vi "test_wpt_sim.vi"() -> ()   [LabVIEW 2019]
uses:
  Ctrl/waypoint_buf.ctl
panel:
  out "size(s)":i32=8
  out "XY Graph":cluster{cluster{dbl, dbl}[]}[](graph)=[{[{7.857142857142858, 2.6530612244897958}]}, {[{-1.0, 1.5}, {-0.9042553191489362, 1.5319148936170213}, {-0.8085106382978724, 1.5638297872340425}, {-0.7127659574468085, 1.5957446808510638}, {-0.6170212765957447, 1.627659574468085}, {-0.5212765957446809, 1.6595744680851063}, {-0.42553191489361697, 1.6914893617021276}, {-0.32978723404255317, 1.7234042553191489}, {-0.23404255319148937, 1.7553191489361701}, {-0.13829787234042556, 1.7872340425531914}, {-0.042553191489361764, 1.8191489361702127}, {0.05319148936170204, 1.851063829787234}, {0.14893617021276606, 1.8829787234042552}, {0.24468085106382986, 1.9148936170212765}, {0.34042553191489366, 1.9468085106382977}, {0.43617021276595747, 1.978723404255319}, {0.5319148936170213, 2.0106382978723403}, {0.6276595744680851, 2.0425531914893615}, {0.7234042553191489, 2.074468085106383}, {0.8191489361702127, 2.106382978723404}, {0.9148936170212765, 2.1382978723404253}, {1.0106382978723403, 2.1702127659574466}, {1.106382978723404, 2.202127659574468}, {1.2021276595744679, 2.234042553191489}, {1.2978723404255321, 2.2659574468085104}, {1.393617021276596, 2.297872340425532}, {1.4893617021276597, 2.329787234042553}, {1.5851063829787235, 2.3617021276595747}, {1.6808510638297873, 2.3936170212765955}, {1.7765957446808511, 2.425531914893617}, {1.872340425531915, 2.457446808510638}, {1.9680851063829787, 2.4893617021276597}, {2.0638297872340425, 2.5212765957446805}, {2.1595744680851063, 2.5531914893617023}, {2.25531914893617, 2.585106382978723}, {2.351063829787234, 2.617021276595745}, {2.4468085106382977, 2.6489361702127656}, {2.5425531914893615, 2.6808510638297873}, {2.6382978723404253, 2.712765957446808}, {2.734042553191489, 2.74468085106383}, {2.829787234042553, 2.7765957446808507}, {2.925531914893617, 2.8085106382978724}, {3.0212765957446805, 2.840425531914893}, {3.117021276595745, 2.872340425531915}, {3.212765957446808, 2.9042553191489358}, {3.3085106382978724, 2.9361702127659575}, {3.4042553191489358, 2.9680851063829783}, {3.5, 3.0}, {3.59375, 2.96875}, {3.6875, 2.9375}, {3.78125, 2.90625}, {3.875, 2.875}, {3.96875, 2.84375}, {4.0625, 2.8125}, {4.15625, 2.78125}, {4.25, 2.75}, {4.34375, 2.71875}, {4.4375, 2.6875}, {4.53125, 2.65625}, {4.625, 2.625}, {4.71875, 2.59375}, {4.8125, 2.5625}, {4.90625, 2.53125}, {5.0, 2.5}, {5.096153846153846, 2.5288461538461537}, {5.1923076923076925, 2.5576923076923075}, {5.288461538461538, 2.5865384615384617}, {5.384615384615385, 2.6153846153846154}, {5.480769230769231, 2.644230769230769}, {5.576923076923077, 2.673076923076923}, {5.673076923076923, 2.701923076923077}, {5.769230769230769, 2.730769230769231}, {5.865384615384615, 2.7596153846153846}, {5.961538461538462, 2.7884615384615383}, {6.0576923076923075, 2.8173076923076925}, {6.153846153846154, 2.8461538461538463}, {6.25, 2.875}, {6.346153846153847, 2.9038461538461537}, {6.4423076923076925, 2.9326923076923075}, {6.538461538461538, 2.9615384615384617}, {6.634615384615385, 2.9903846153846154}, {6.730769230769231, 3.019230769230769}, {6.826923076923077, 3.0480769230769234}, {6.923076923076923, 3.076923076923077}, {7.019230769230769, 3.105769230769231}, {7.115384615384615, 3.1346153846153846}, {7.211538461538462, 3.1634615384615383}, {7.307692307692308, 3.1923076923076925}, {7.403846153846154, 3.2211538461538463}, {7.5, 3.25}, {7.596153846153847, 3.2788461538461537}, {7.6923076923076925, 3.3076923076923075}, {7.788461538461538, 3.3365384615384617}, {7.884615384615385, 3.3653846153846154}, {7.980769230769231, 3.394230769230769}, {8.076923076923077, 3.4230769230769234}, {8.173076923076923, 3.451923076923077}, {8.26923076923077, 3.480769230769231}, {8.365384615384615, 3.5096153846153846}, {8.461538461538462, 3.5384615384615383}, {8.557692307692308, 3.5673076923076925}, {8.653846153846153, 3.5961538461538463}, {8.75, 3.625}, {8.846153846153847, 3.653846153846154}, {8.942307692307693, 3.6826923076923075}, {9.038461538461538, 3.7115384615384617}, {9.134615384615385, 3.7403846153846154}, {9.23076923076923, 3.769230769230769}, {9.326923076923077, 3.7980769230769234}, {9.423076923076923, 3.826923076923077}, {9.51923076923077, 3.855769230769231}, {9.615384615384617, 3.8846153846153846}, {9.711538461538462, 3.9134615384615383}, {9.807692307692308, 3.9423076923076925}, {9.903846153846153, 3.9711538461538463}, {10.0, 4.0}, {10.06, 3.92}, {10.12, 3.84}, {10.18, 3.76}, {10.24, 3.68}, {10.3, 3.6}, {10.36, 3.52}, {10.42, 3.44}, {10.48, 3.36}, {10.54, 3.2800000000000002}, {10.6, 3.2}, {10.66, 3.12}, {10.72, 3.04}, {10.78, 2.96}, {10.84, 2.88}, {10.9, 2.8}, {10.96, 2.7199999999999998}, {11.02, 2.6399999999999997}, {11.08, 2.56}, {11.14, 2.48}, {11.2, 2.4}, {11.26, 2.3200000000000003}, {11.32, 2.24}, {11.379999999999999, 2.16}, {11.44, 2.08}, {11.5, 2.0}, {11.56, 1.92}, {11.62, 1.8399999999999999}, {11.68, 1.7599999999999998}, {11.74, 1.6800000000000002}, {11.8, 1.6}, {11.86, 1.52}, {11.92, 1.44}, {11.98, 1.3599999999999999}, {12.04, 1.2799999999999998}, {12.1, 1.1999999999999997}, {12.16, 1.12}, {12.219999999999999, 1.04}, {12.28, 0.96}, {12.34, 0.8799999999999999}, {12.4, 0.7999999999999998}, {12.46, 0.7199999999999998}, {12.52, 0.6400000000000001}, {12.58, 0.56}, {12.64, 0.48}, {12.7, 0.3999999999999999}, {12.76, 0.31999999999999984}, {12.82, 0.23999999999999977}, {12.879999999999999, 0.16000000000000014}, {12.94, 0.08000000000000007}, {13.0, 0.0}, {12.928571428571429, -0.07142857142857142}, {12.857142857142858, -0.14285714285714285}, {12.785714285714286, -0.21428571428571427}, {12.714285714285714, -0.2857142857142857}, {12.642857142857142, -0.3571428571428571}, {12.571428571428571, -0.42857142857142855}, {12.5, -0.5}, {12.428571428571429, -0.5714285714285714}, {12.357142857142858, -0.6428571428571428}, {12.285714285714286, -0.7142857142857142}, {12.214285714285714, -0.7857142857142857}, {12.142857142857142, -0.8571428571428571}, {12.071428571428571, -0.9285714285714285}, {12.0, -1.0}, {11.928571428571429, -1.0714285714285714}, {11.857142857142858, -1.1428571428571428}, {11.785714285714286, -1.2142857142857142}, {11.714285714285715, -1.2857142857142856}, {11.642857142857142, -1.357142857142857}, {11.571428571428571, -1.4285714285714284}, {11.5, -1.5}, {11.428571428571429, -1.5714285714285714}, {11.357142857142858, -1.6428571428571428}, {11.285714285714286, -1.7142857142857142}, {11.214285714285715, -1.7857142857142856}, {11.142857142857142, -1.857142857142857}, {11.071428571428571, -1.9285714285714284}, {11.0, -2.0}, {10.928571428571429, -2.071428571428571}, {10.857142857142858, -2.142857142857143}, {10.785714285714286, -2.214285714285714}, {10.714285714285715, -2.2857142857142856}, {10.642857142857142, -2.357142857142857}, {10.571428571428571, -2.4285714285714284}, {10.5, -2.5}, {10.428571428571429, -2.571428571428571}, {10.357142857142858, -2.642857142857143}, {10.285714285714286, -2.714285714285714}, {10.214285714285715, -2.7857142857142856}, {10.142857142857142, -2.8571428571428568}, {10.071428571428571, -2.9285714285714284}, {10.0, -3.0}, {9.901960784313726, -3.019607843137255}, {9.803921568627452, -3.0392156862745097}, {9.705882352941176, -3.0588235294117645}, {9.607843137254902, -3.0784313725490198}, {9.509803921568627, -3.0980392156862746}, {9.411764705882353, -3.1176470588235294}, {9.313725490196079, -3.1372549019607843}, {9.215686274509803, -3.156862745098039}, {9.117647058823529, -3.176470588235294}, {9.019607843137255, -3.196078431372549}, {8.92156862745098, -3.215686274509804}, {8.823529411764707, -3.235294117647059}, {8.725490196078432, -3.2549019607843137}, {8.627450980392156, -3.2745098039215685}, {8.529411764705882, -3.2941176470588234}, {8.431372549019608, -3.313725490196078}, {8.333333333333334, -3.3333333333333335}, {8.235294117647058, -3.3529411764705883}, {8.137254901960784, -3.372549019607843}, {8.03921568627451, -3.392156862745098}, {7.9411764705882355, -3.411764705882353}, {7.843137254901961, -3.431372549019608}, {7.745098039215686, -3.450980392156863}, {7.647058823529411, -3.4705882352941178}, {7.549019607843137, -3.4901960784313726}, {7.450980392156863, -3.5098039215686274}, {7.352941176470589, -3.5294117647058822}, {7.254901960784314, -3.549019607843137}, {7.156862745098039, -3.568627450980392}, {7.0588235294117645, -3.588235294117647}, {6.96078431372549, -3.607843137254902}, {6.862745098039216, -3.627450980392157}, {6.764705882352941, -3.6470588235294117}, {6.666666666666666, -3.6666666666666665}, {6.568627450980392, -3.686274509803922}, {6.470588235294118, -3.7058823529411766}, {6.372549019607844, -3.7254901960784315}, {6.2745098039215685, -3.7450980392156863}, {6.176470588235294, -3.764705882352941}, {6.078431372549019, -3.784313725490196}, {5.980392156862745, -3.803921568627451}, {5.882352941176471, -3.8235294117647056}, {5.784313725490196, -3.843137254901961}, {5.686274509803922, -3.8627450980392157}, {5.588235294117647, -3.8823529411764706}, {5.490196078431373, -3.9019607843137254}, {5.392156862745098, -3.9215686274509802}, {5.294117647058823, -3.9411764705882355}, {5.196078431372549, -3.9607843137254903}, {5.098039215686274, -3.980392156862745}, {5.0, -4.0}, {4.90625, -3.96875}, {4.8125, -3.9375}, {4.71875, -3.90625}, {4.625, -3.875}, {4.53125, -3.84375}, {4.4375, -3.8125}, {4.34375, -3.78125}, {4.25, -3.75}, {4.15625, -3.71875}, {4.0625, -3.6875}, {3.96875, -3.65625}, {3.875, -3.625}, {3.78125, -3.59375}, {3.6875, -3.5625}, {3.59375, -3.53125}, {3.5, -3.5}, {3.40625, -3.46875}, {3.3125, -3.4375}, {3.21875, -3.40625}, {3.125, -3.375}, {3.03125, -3.34375}, {2.9375, -3.3125}, {2.84375, -3.28125}, {2.75, -3.25}, {2.65625, -3.21875}, {2.5625, -3.1875}, {2.46875, -3.15625}, {2.375, -3.125}, {2.28125, -3.09375}, {2.1875, -3.0625}, {2.09375, -3.03125}, {2.0, -3.0}, {1.9, -3.0166666666666666}, {1.8, -3.033333333333333}, {1.7, -3.05}, {1.6, -3.066666666666667}, {1.5, -3.0833333333333335}, {1.4, -3.1}, {1.2999999999999998, -3.1166666666666667}, {1.2, -3.1333333333333333}, {1.1, -3.15}, {1.0, -3.1666666666666665}, {0.8999999999999999, -3.183333333333333}, {0.7999999999999998, -3.2}, {0.7, -3.216666666666667}, {0.5999999999999999, -3.2333333333333334}, {0.5, -3.25}, {0.3999999999999999, -3.2666666666666666}, {0.2999999999999998, -3.283333333333333}, {0.19999999999999996, -3.3}, {0.09999999999999987, -3.3166666666666664}, {0.0, -3.3333333333333335}, {-0.10000000000000009, -3.35}, {-0.20000000000000018, -3.3666666666666667}, {-0.30000000000000027, -3.3833333333333333}, {-0.40000000000000036, -3.4}, {-0.5, -3.4166666666666665}, {-0.6000000000000001, -3.4333333333333336}, {-0.7000000000000002, -3.45}, {-0.8000000000000003, -3.466666666666667}, {-0.9000000000000004, -3.4833333333333334}, {-1.0, -3.5}, {-1.0555555555555556, -3.4166666666666665}, {-1.1111111111111112, -3.3333333333333335}, {-1.1666666666666667, -3.25}, {-1.2222222222222223, -3.1666666666666665}, {-1.2777777777777777, -3.0833333333333335}, {-1.3333333333333333, -3.0}, {-1.3888888888888888, -2.916666666666667}, {-1.4444444444444444, -2.8333333333333335}, {-1.5, -2.75}, {-1.5555555555555556, -2.666666666666667}, {-1.6111111111111112, -2.5833333333333335}, {-1.6666666666666665, -2.5}, {-1.7222222222222223, -2.416666666666667}, {-1.7777777777777777, -2.3333333333333335}, {-1.8333333333333333, -2.25}, {-1.8888888888888888, -2.166666666666667}, {-1.9444444444444444, -2.0833333333333335}, {-2.0, -2.0}, {-1.96875, -1.90625}, {-1.9375, -1.8125}, {-1.90625, -1.71875}, {-1.875, -1.625}, {-1.84375, -1.53125}, {-1.8125, -1.4375}, {-1.78125, -1.34375}, {-1.75, -1.25}, {-1.71875, -1.15625}, {-1.6875, -1.0625}, {-1.65625, -0.96875}, {-1.625, -0.875}, {-1.59375, -0.78125}, {-1.5625, -0.6875}, {-1.53125, -0.59375}, {-1.5, -0.5}, {-1.46875, -0.40625}, {-1.4375, -0.3125}, {-1.40625, -0.21875}, {-1.375, -0.125}, {-1.34375, -0.03125}, {-1.3125, 0.0625}, {-1.28125, 0.15625}, {-1.25, 0.25}, {-1.21875, 0.34375}, {-1.1875, 0.4375}, {-1.15625, 0.53125}, {-1.125, 0.625}, {-1.09375, 0.71875}, {-1.0625, 0.8125}, {-1.03125, 0.90625}]}, {[{5.865384615384615, 2.7596153846153846}, {5.961538461538462, 2.7884615384615383}, {6.0576923076923075, 2.8173076923076925}, {6.153846153846154, 2.8461538461538463}, {6.25, 2.875}, {6.346153846153847, 2.9038461538461537}, {6.4423076923076925, 2.9326923076923075}, {6.538461538461538, 2.9615384615384617}, {6.634615384615385, 2.9903846153846154}, {6.730769230769231, 3.019230769230769}, {6.826923076923077, 3.0480769230769234}, {6.923076923076923, 3.076923076923077}, {7.019230769230769, 3.105769230769231}, {7.115384615384615, 3.1346153846153846}, {7.211538461538462, 3.1634615384615383}, {7.307692307692308, 3.1923076923076925}, {7.403846153846154, 3.2211538461538463}, {7.5, 3.25}, {7.596153846153847, 3.2788461538461537}, {7.6923076923076925, 3.3076923076923075}, {7.788461538461538, 3.3365384615384617}, {7.884615384615385, 3.3653846153846154}, {7.980769230769231, 3.394230769230769}, {8.076923076923077, 3.4230769230769234}, {8.173076923076923, 3.451923076923077}, {8.26923076923077, 3.480769230769231}, {8.365384615384615, 3.5096153846153846}, {8.461538461538462, 3.5384615384615383}, {8.557692307692308, 3.5673076923076925}, {8.653846153846153, 3.5961538461538463}, {8.75, 3.625}, {8.846153846153847, 3.653846153846154}, {8.942307692307693, 3.6826923076923075}, {9.038461538461538, 3.7115384615384617}, {9.134615384615385, 3.7403846153846154}, {9.23076923076923, 3.769230769230769}, {9.326923076923077, 3.7980769230769234}, {9.423076923076923, 3.826923076923077}]}, {[{7.857142857142858, 4.653061224489796}, {8.05317713780198, 4.643430677834189}, {8.247323501175114, 4.614631785296257}, {8.437712211651782, 4.566941895954214}, {8.622509721873037, 4.500820289512369}, {8.799936330794853, 4.416903753186506}, {8.968283323182062, 4.3160004490948864}, {9.125929425470149, 4.1990821312152695}, {9.271356419515953, 4.067274786862891}, {9.403163763868331, 3.9218477928170867}, {9.520082081747947, 3.764201690529}, {9.620985385839568, 3.5958546981417916}, {9.704901922165432, 3.4184280892199754}, {9.771023528607275, 3.2336305789987203}, {9.818713417949319, 3.0432418685220526}, {9.847512310487252, 2.8490955051489175}, {9.857142857142858, 2.6530612244897958}, {9.847512310487252, 2.4570269438306744}, {9.818713417949319, 2.2628805804575394}, {9.771023528607275, 2.0724918699808716}, {9.704901922165432, 1.8876943597596163}, {9.620985385839568, 1.7102677508378004}, {9.52008208174795, 1.5419207584505918}, {9.403163763868331, 1.384274656162505}, {9.271356419515953, 1.2388476621167008}, {9.125929425470149, 1.1070403177643218}, {8.968283323182062, 0.9901219998847051}, {8.799936330794853, 0.8892186957930859}, {8.622509721873037, 0.8053021594672223}, {8.437712211651782, 0.7391805530253781}, {8.247323501175115, 0.6914906636833349}, {8.05317713780198, 0.6626917711454021}, {7.857142857142858, 0.6530612244897958}, {7.661108576483737, 0.6626917711454019}, {7.466962213110601, 0.6914906636833349}, {7.2765735026339335, 0.7391805530253779}, {7.091775992412678, 0.8053021594672221}, {6.914349383490863, 0.8892186957930857}, {6.746002391103653, 0.9901219998847048}, {6.588356288815567, 1.1070403177643215}, {6.442929294769763, 1.2388476621167004}, {6.311121950417384, 1.384274656162504}, {6.194203632537767, 1.5419207584505914}, {6.093300328446148, 1.7102677508378}, {6.009383792120285, 1.8876943597596152}, {5.9432621856784404, 2.0724918699808708}, {5.895572296336397, 2.2628805804575385}, {5.866773403798463, 2.457026943830675}, {5.857142857142858, 2.6530612244897953}, {5.866773403798463, 2.8490955051489157}, {5.895572296336397, 3.0432418685220526}, {5.94326218567844, 3.23363057899872}, {6.009383792120285, 3.418428089219976}, {6.093300328446148, 3.5958546981417907}, {6.194203632537767, 3.7642016905289992}, {6.311121950417384, 3.921847792817087}, {6.442929294769762, 4.067274786862891}, {6.588356288815566, 4.199082131215269}, {6.746002391103653, 4.3160004490948864}, {6.914349383490862, 4.416903753186506}, {7.091775992412677, 4.500820289512369}, {7.276573502633933, 4.566941895954214}, {7.4669622131106, 4.614631785296257}, {7.661108576483737, 4.643430677834189}, {7.857142857142857, 4.653061224489796}]}, {[{7.644230769230769, 3.293269230769231}, {7.857142857142858, 2.6530612244897958}]}, {[{9.403163763868331, 3.9218477928170867}]}, {[]}, {[{-1.0, 1.5}, {3.5, 3.0}, {5.0, 2.5}, {10.0, 4.0}, {13.0, 0.0}, {10.0, -3.0}, {5.0, -4.0}, {2.0, -3.0}, {-1.0, -3.5}, {-2.0, -2.0}, {-1.0, 1.0}]}]
  in  "stop":bool=TRUE
  in  "agv":cluster{dbl, dbl}={7.857142857142858, 2.6530612244897958} {"?" scale=-5.0..15.0; "?" scale=-5.0..10.0}
  in  "way point":cluster{dbl, dbl}[](array[cluster])=[{-1.0, 1.5}, {3.5, 3.0}, {5.0, 2.5}, {10.0, 4.0}, {13.0, 0.0}, {10.0, -3.0}, {5.0, -4.0}, {2.0, -3.0}, {-1.0, -3.5}, {-2.0, -2.0}, {-1.0, 1.0}]
  in  "lookahed cfg in":T1={"lookahead pt n"=64.0, "lookahead distance "=2.0}
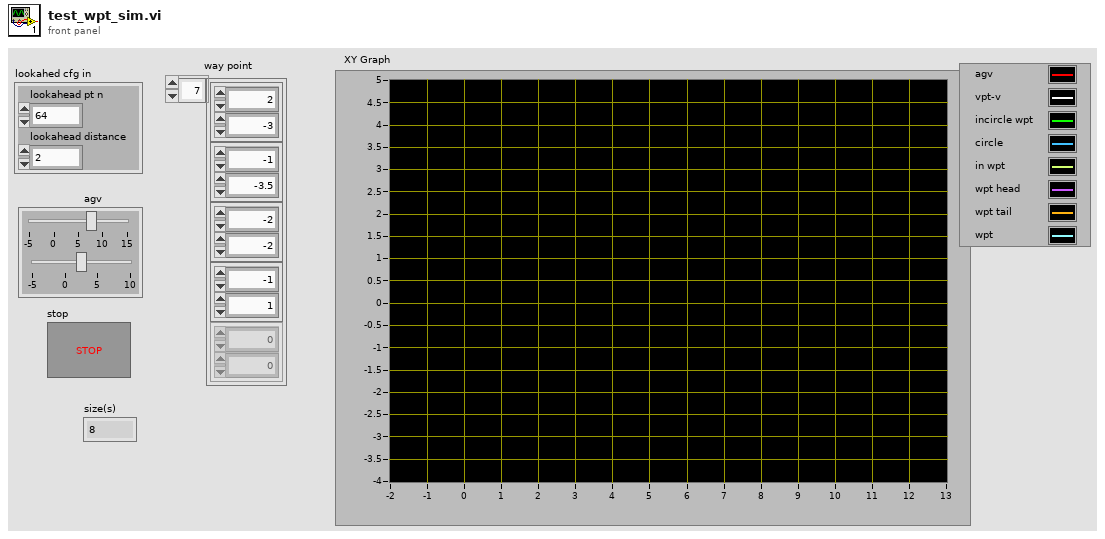
[diagram p1: front panel]
types:
  T1 = cluster{"lookahead pt n":dbl, "lookahead distance ":dbl}
  T2 = typedef "waypoint_buf.ctl" = enum16{"clear", "write", "read"}
  T3 = cluster{"incircle wpt":cluster{dbl, dbl}[], "agv circle":cluster{dbl, dbl}[], "offset":cluster{dbl, dbl}[], "lookahead":cluster{"x":dbl, "y":dbl}[], "looktail":cluster{"x":dbl, "y":dbl}[]}
  T4 = cluster{"waypoint out":cluster{"x":dbl, "y":dbl}[]}
  T5 = cluster{"waypoint out":cluster{"x":dbl, "y":dbl}[]}[]
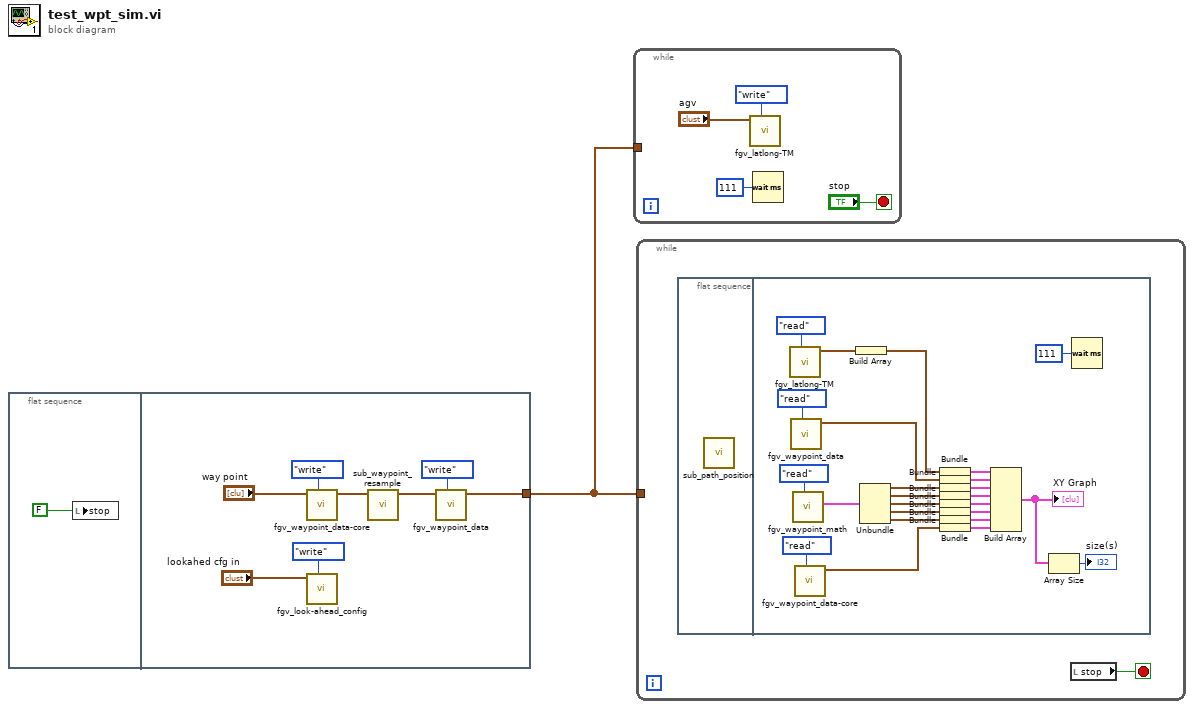
[diagram p0: block diagram]
diagram:
  n1 = flat-sequence {
    tunnel: [w3] -> w1
    frame #0 {
      n2 = local write "stop"(FALSE ("stop")) -> ()
    }
    frame #1 {
      n3 = call "fgv_waypoint_data-core.vi"("cmd"=waypoint_buf."write", "ori-waypoint"="way point") -> ("waypoint out"=w5:cluster{"x":dbl, "y":dbl}[])  [unwired: 9 in]
      n4 = call "fgv_look-ahead_config.vi"("cmd"=enum16{"read", "write"}."write", "lookahed cfg in"="lookahed cfg in") -> ()  [unwired: 9 in, 1 out]
      n5 = call "sub_waypoint_resample.vi"("line point"=w5) -> ("interpolate 1d array"=w4:cluster{dbl, dbl}[])  [unwired: 9 in, 1 out]
      n6 = call "fgv_waypoint_data.vi"("cmd"=waypoint_buf."write", "waypoint in"=w4) -> ("waypoint out"=w3:cluster{"x":dbl, "y":dbl}[])  [unwired: 7 in, 2 out]
    }
  }
  n7 = while {
    tunnel: w1 -> [_]
    stop <- "stop" stop-if-true
    n8 = call "fgv_latlong-TM.vi"("cmd"=enum16{"write", "read"}."write", "tm"="agv") -> ()  [unwired: 8 in, 2 out]
    n9 = Wait (ms)(milliseconds to wait=u32 111) -> ()  [unwired: 1 out]
  }
  n10 = while {
    tunnel: w1 -> [_]
    stop <- w15 stop-if-true
    n11 = flat-sequence {
      frame #0 {
        n12 = call "sub_path_position.vi"() -> ()  [unwired: 12 in]
      }
      frame #1 {
        n13 = call "fgv_latlong-TM.vi"("cmd"=enum16{"write", "read"}."read") -> ("tm out"=w37:cluster{dbl, dbl})  [unwired: 9 in, 1 out]
        n14 = call "fgv_waypoint_data.vi"("cmd"=waypoint_buf."read") -> ("waypoint out"=w20:cluster{"x":dbl, "y":dbl}[])  [unwired: 8 in, 2 out]
        n15 = call "fgv_waypoint_math.vi"("cmd"=waypoint_buf."read") -> ("wpt data"=w39:T3)  [unwired: 9 in, 1 out]
        n16 = call "fgv_waypoint_data-core.vi"("cmd"=waypoint_buf."read") -> ("waypoint out"=w23:cluster{"x":dbl, "y":dbl}[])  [unwired: 10 in]
        n17 = Build Array(w37) -> (w29:cluster{dbl, dbl}[])
        n18 = Unbundle(w39) -> ("incircle wpt"=w28:cluster{dbl, dbl}[], "agv circle"=w27:cluster{dbl, dbl}[], "offset"=w26:cluster{dbl, dbl}[], "lookahead"=w25:cluster{"x":dbl, "y":dbl}[], "looktail"=w24:cluster{"x":dbl, "y":dbl}[])
        n19 = Bundle(w29) -> (w22:cluster{cluster{dbl, dbl}[]})  [unwired: 1 in]
        n20 = Bundle("waypoint out"=w20) -> (w19:T4)  [unwired: 1 in]
        n21 = Bundle("incircle wpt"=w28) -> (w30:cluster{"incircle wpt":cluster{dbl, dbl}[]})  [unwired: 1 in]
        n22 = Bundle("agv circle"=w27) -> (w31:cluster{"agv circle":cluster{dbl, dbl}[]})  [unwired: 1 in]
        n23 = Bundle("offset"=w26) -> (w32:cluster{"offset":cluster{dbl, dbl}[]})  [unwired: 1 in]
        n24 = Bundle("lookahead"=w25) -> (w33:cluster{"lookahead":cluster{"x":dbl, "y":dbl}[]})  [unwired: 1 in]
        n25 = Bundle("looktail"=w24) -> (w34:cluster{"looktail":cluster{"x":dbl, "y":dbl}[]})  [unwired: 1 in]
        n26 = Bundle("waypoint out"=w23) -> (w35:T4)  [unwired: 1 in]
        n27 = Build Array(w22, w19, w30, w31, w32, w33, w34, w35) -> (w18:T5)
        "XY Graph" <- w18
        n28 = Array Size(array=w18) -> (size(s)=→"size(s)":i32)
        n29 = Wait (ms)(milliseconds to wait=u32 111) -> ()  [unwired: 1 out]
      }
    }
    n30 = local read "stop"() -> (w15:bool)
  }
